vi "FGV_Setup.vi"(8 "Type":enum16{"Read", "Write"}(ring), 11 "InSetup":T3={"AquisitionParameters"={"SampleRate"=10000.0, "BufferSize"=512, "Channels"="cDAQ1Mod1/ai0:3"}, "SoundFormat"={"sample rate (S/s)"=22050.0, "number of channels"=2, "bits per sample"=16}, "Signal type"=enum."Sine Wave", "Amplitude"=1.0, "AudioBuffer"=0, "ChannelBounds"=[], "MasterOffset"=0.0} {"MasterOffset" scale=10.0..10000.0; "Amplitude" format="%0.2f"}) -> (3 "OutSetup":T3={"AquisitionParameters"={"SampleRate"=10000.0, "BufferSize"=512, "Channels"="cDAQ1Mod1/ai0:3"}, "SoundFormat"={"sample rate (S/s)"=22050.0, "number of channels"=2, "bits per sample"=16}, "Signal type"=enum."Sine Wave", "Amplitude"=1.0, "AudioBuffer"=0, "ChannelBounds"=[], "MasterOffset"=0.0} {"MasterOffset" scale=10.0..10000.0; "Amplitude" format="%0.2f"})   [LabVIEW 2024]
uses:
  dacAquisition/#AquisitionParameter.ctl
  <vilib>/sound2/lvsound2.llb/Sound Data Format.ctl
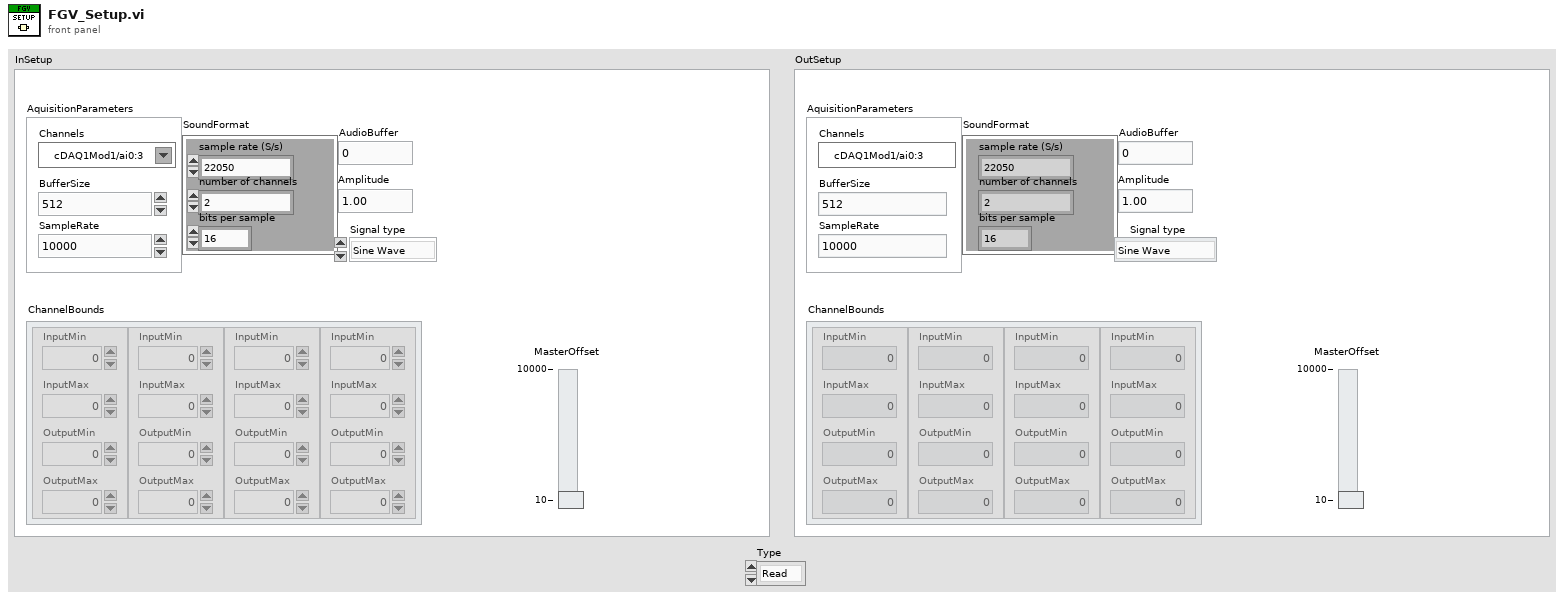
[diagram p1: front panel]
types:
  T1 = typedef "#AquisitionParameter.ctl" = cluster{"SampleRate":dbl, "BufferSize":i32, "Channels":tag}
  T2 = typedef "Sound Data Format.ctl" = cluster{"sample rate (S/s)":dbl, "number of channels":i32, "bits per sample":i32}
  T3 = cluster{"AquisitionParameters":T1, "SoundFormat":T2, "Signal type":enum16{"Sine Wave", "Triangle Wave", "Square Wave", "Sawtooth Wave"}, "Amplitude":dbl, "AudioBuffer":i32, "ChannelBounds":cluster{"InputMin":dbl, "InputMax":dbl, "OutputMin":dbl, "OutputMax":dbl}[], "MasterOffset":dbl}
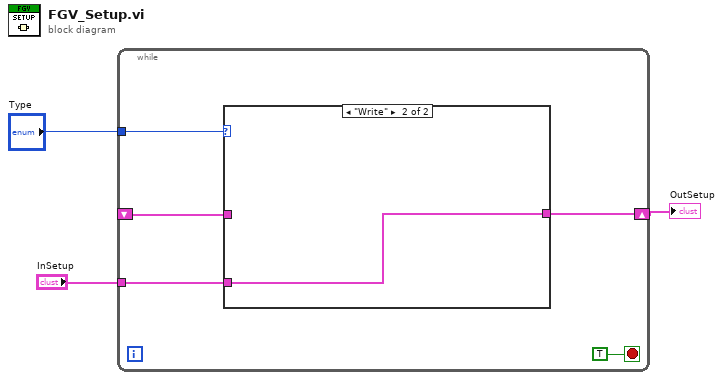
[diagram p0: block diagram]
diagram:
  n1 = while {
    tunnel: "Type" -> [w7]
    shift-right: [w5] -> w1
    shift-left: _ -> [w6]
    tunnel: "InSetup" -> [w4]
    stop <- TRUE stop-if-true
    n2 = case shown="\"Write\"" w7 {
      tunnel: w6 -> [w9 _]
      tunnel: [w9 w10] -> w5
      tunnel: w4 -> [_ w10]
      frame "Read" {
      }
      frame "Write" {
      }
    }
  }
  "OutSetup" <- w1
